vi "Close.vi"(8 "error in":errorcluster, 11 "Red-y Read Write CFG in":refnum<class "Red-y Pressure Control CFG Simulated.lvclass">) -> (0 "error out":errorcluster, 3 "Red-y Read Write CFG out":refnum<class "Red-y Pressure Control CFG Simulated.lvclass">)   [LabVIEW 2023, in "Red-y Pressure Control CFG Simulated.lvclass"]
uses:
  Red-y Pressure Control CFG Simulated.lvclass
  Pressure Control CFG/Red-y Pressure Control CFG.lvclass
  Red-y Pressure Control CFG Simulated.lvclass/Red-y Pressure Control CFG Simulated.ctl
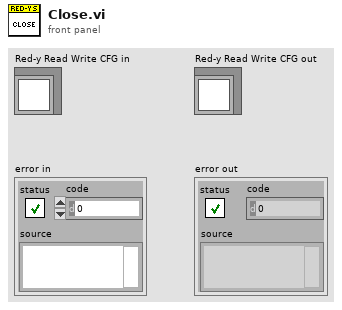
[diagram p1: front panel]
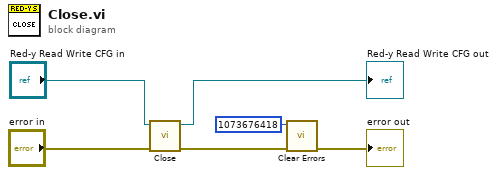
[diagram p0: block diagram]
diagram:
  n1 = call-parent "Close.vi"("error in"="error in", "Red-y Read Write CFG in"="Red-y Read Write CFG in") -> ("error out"=w6:errorcluster, "Red-y Read Write CFG out"=→"Red-y Read Write CFG out":refnum<class "Red-y Pressure Control CFG Simulated.lvclass">)  [unwired: 8 in]
  n2 = call <vilib>:"Clear Errors.vi"("error in (no error)"=w6, "specific error code to clear (0: all)"=1073676418) -> ("error out"=→"error out":errorcluster)  [unwired: 4 in, 1 out]
